vi "Get_Indicies_of_Crossconnected_Points-1.vi"(2 "[IN] Index of point":i32, 3 "[IN] Indicies of Cross\nconnected Points":i32[](array[numeric])) -> (0 "[OUT] Column index":i32, 1 "[OUT] Row index":i32)   [LabVIEW 2013]
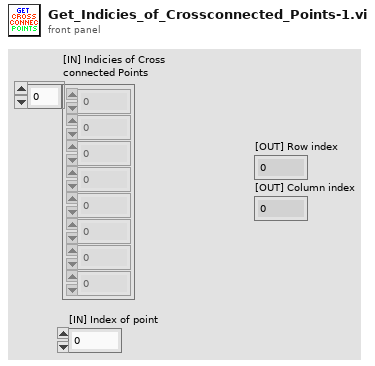
[diagram p1: front panel]
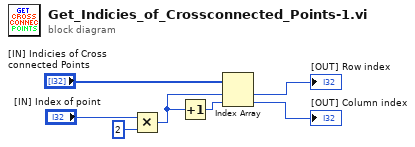
[diagram p0: block diagram]
diagram:
  n1 = Multiply(x="[IN] Index of point", y=2) -> (x*y=w4:i32)
  n2 = Increment(x=w4) -> (x+1=w3:i32)
  n3 = Index Array(array="[IN] Indicies of Cross\nconnected Points", index #1=w4, index #2=w3) -> (element #1=→"[OUT] Row index":i32, element #2=→"[OUT] Column index":i32)
